vi "UI Page Disply_Error Occur.vi"(8 "error in (no error)":errorcluster, 10 "Tab Main":refnum<vi>, 11 "MPC_Laser Marked in":refnum<class "MPC_Laser Marked.lvclass">) -> (0 "error out":errorcluster, 3 "MPC_Laser Marked out":refnum<class "MPC_Laser Marked.lvclass">)   [LabVIEW 2019, in "MPC_Laser Marked.lvclass"]
uses:
  MPC_Laser Marked.lvclass
  Function/IO Folder/IO_VI/IOCtrl/Ctrl/DMC1000B_1 SelectOutput.ctl
  Main Class.lvclass
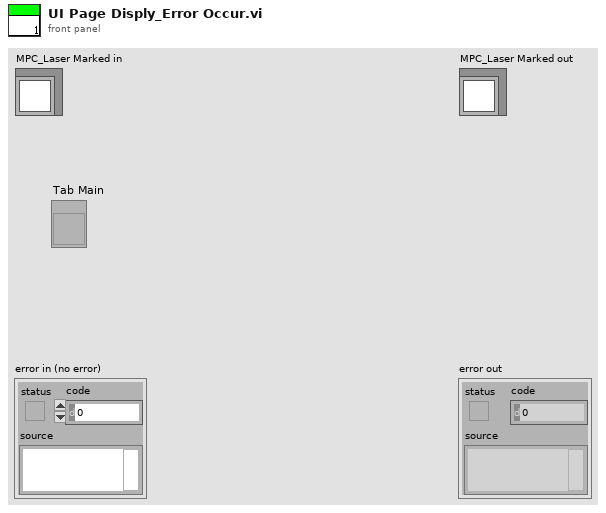
[diagram p1: front panel]
types:
  T1 = typedef "DMC1000B_1 SelectOutput.ctl" = enum16{"M_Out0預備", "M_OUT01蜂鳴器", "M_OUT02紅燈", "M_OUT03綠燈", "M_OUT04黃燈", "M_OUT05上頂固定位氣缸電磁閥", "M_OUT06到料阻擋氣缸電磁閥", "M_OUT07向前機台發出要料#1信號", "M_OUT08向前機台發出要料#2信號", "M_OUT09向後機台發出有料#3信號", "M_OUT10向後機台發出有料#4信號", "M_OUT11接駁台馬達啟動開/關", "M_OUT12接駁台馬達慢速", "M_OUT13抽風機開/關", "M_OUT14上視覺上光源", "M_OUT15DC吹風扇開/關", "M_OUT16Z軸煞車釋放", "M_OUT17", "M_OUT18", "M_OUT19", "M_OUT20", "M_OUT21", "M_OUT22", "M_OUT23", "M_OUT24", "M_OUT25第一軸SEVON1伺服使能信號", "M_OUT26第二軸SEVON2伺服使能信號", "M_OUT27第三軸SEVON3伺服使能信號"}
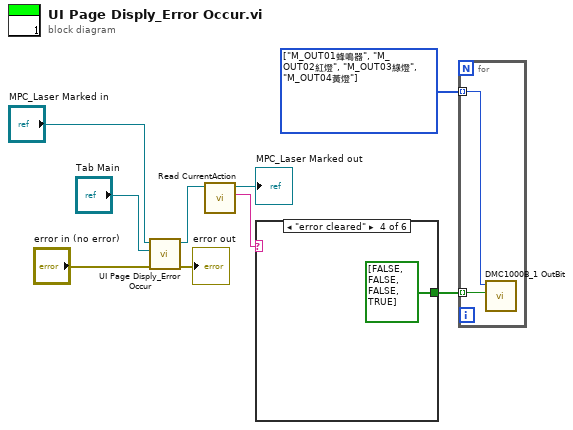
[diagram p0: block diagram]
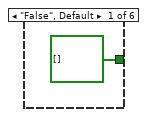
[diagram p2: hidden frame]
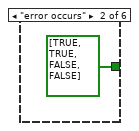
[diagram p3: hidden frame]
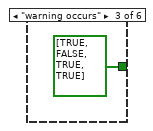
[diagram p4: hidden frame]
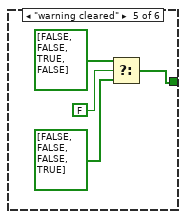
[diagram p5: hidden frame]
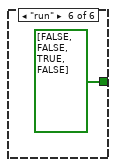
[diagram p6: hidden frame]
diagram:
  w1 = T1[] [enum."M_OUT01蜂鳴器", enum."M_OUT02紅燈", enum."M_OUT03綠燈", enum."M_OUT04黃燈"] items=["M_Out0預備", "M_OUT01蜂鳴器", "M_OUT02紅燈", "M_OUT03綠燈", "M_OUT04黃燈", "M_OUT05上頂固定位氣缸電磁閥", "M_OUT06到料阻擋氣缸電磁閥", "M_OUT07向前機台發出要料#1信號", "M_OUT08向前機台發出要料#2信號", "M_OUT09向後機台發出有料#3信號", "M_OUT10向後機台發出有料#4信號", "M_OUT11接駁台馬達啟動開/關", "M_OUT12接駁台馬達慢速", "M_OUT13抽風機開/關", "M_OUT14上視覺上光源", "M_OUT15DC吹風扇開/關", "M_OUT16Z軸煞車釋放", "M_OUT17", "M_OUT18", "M_OUT19", "M_OUT20", "M_OUT21", "M_OUT22", "M_OUT23", "M_OUT24", "M_OUT25第一軸SEVON1伺服使能信號", "M_OUT26第二軸SEVON2伺服使能信號", "M_OUT27第三軸SEVON3伺服使能信號"]
  n1 = call-parent "UI Page Disply_Error Occur.vi"("error in (no error)"="error in (no error)", "Tab Main"="Tab Main", "Main Class in"="MPC_Laser Marked in") -> ("error out"=→"error out":errorcluster, "Main Class out"=w5:refnum<class "MPC_Laser Marked.lvclass">)  [unwired: 7 in]
  n2 = call-dynamic "Read CurrentAction.vi"("Main Process Class in"=w5) -> ("CurrentAction"=w3:string, "Main Process Class out"=→"MPC_Laser Marked out":refnum<class "MPC_Laser Marked.lvclass">)  [unwired: 8 in, 1 out]
  n3 = case shown="\"error cleared\"" w3 {
    tunnel: [bool[] [] bool[] [TRUE, TRUE, FALSE, FALSE] bool[] [TRUE, FALSE, TRUE, TRUE] bool[] [FALSE, FALSE, FALSE, TRUE] w16 bool[] [FALSE, FALSE, TRUE, FALSE]] -> w2
    frame "False", Default {
    }
    frame "error occurs" {
    }
    frame "warning occurs" {
    }
    frame "error cleared" {
    }
    frame "warning cleared" {
      n4 = Select(t=bool[] [FALSE, FALSE, TRUE, FALSE], s=FALSE, f=bool[] [FALSE, FALSE, FALSE, TRUE]) -> (s? t:f=w16:bool[])
    }
    frame "run" {
    }
  }
  n5 = for {
    tunnel: w2 -> [w19] mode=indexing
    tunnel: w1 -> [w20] mode=indexing
    n6 = call "DMC1000B_1 OutBit.vi"("BL"=w19, "IO_Output_1 Select"=w20) -> ()  [unwired: 9 in, 1 out]
  }
